vi "Regenerate STM Link.vi"(7 "IP Address":string, 8 "error in (no error)":errorcluster, 11 "connection info in":T1) -> (0 "error out":errorcluster, 3 "connection info out":T1)   [LabVIEW 2016, in "Assert API Components.lvlib" / "Assert Service.lvlib" / "Assert Service.lvclass"]
uses:
  Assert Service.lvclass
  <vilib>/NI/STM/TCP/TCP Connection Info.ctl
  <vilib>/NI/STM/SubVIs/MetaDataElement.ctl
  <vilib>/NI/STM/TCP/Get Connection Reference (TCP).vi
  <vilib>/NI/STM/TCP/Read Meta Data (TCP Clst).vi
  <vilib>/NI/STM/TCP/Read Meta Data (TCP Ref).vi
  <vilib>/NI/STM/NI STM.lvlib
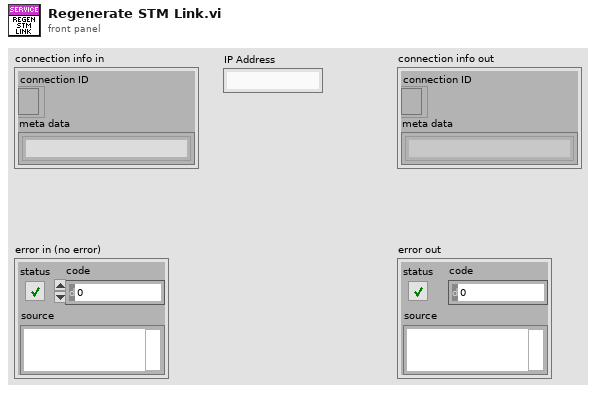
[diagram p1: front panel]
types:
  T1 = typedef "NI STM.lvlib/TCP Connection Info.ctl" = cluster{"connection ID":refnum<k5>, "meta data":T2[]}
  T2 = typedef "NI STM.lvlib/MetaDataElement.ctl" = string
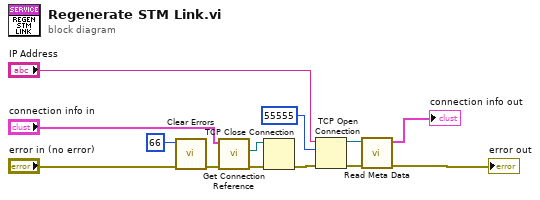
[diagram p0: block diagram]
diagram:
  n1 = call <vilib>:"Clear Errors.vi"("error in (no error)"="error in (no error)", "specific error code to clear (0: all)"=66) -> ("error out"=w11:errorcluster)  [unwired: 4 in, 1 out]
  n2 = call-poly <vilib>:"Get Connection Reference.vi"("error in"=w11, "connection info in"="connection info in") -> ("error out"=w3:errorcluster, "connection ID out"=w2:refnum<k5>)  [unwired: 8 out]
  n3 = TCP Close Connection(connection ID=w2, error in (no error)=w3) -> (error out=w8:errorcluster)  [unwired: 2 out]
  n4 = TCP Open Connection(address="IP Address", remote port or service name=u16 55555 ("remote port"), error in (no error)=w8) -> (connection ID=w6:refnum<k5>, error out=w9:errorcluster)  [unwired: 2 out]
  n5 = call-poly <vilib>:"Read Meta Data.vi"("error in"=w9, "connection ID"=w6) -> ("error out"=→"error out":errorcluster, "connection info out"=→"connection info out":T1)  [unwired: 7 in, 1 out]
